vi "New SPL Calc.vi"(10 "Filtered Signal":dynamicdata(waveform), 11 "Reset":bool) -> (3 "SPL Out":dbl)   [LabVIEW 2020, in "CollectionSupport.lvlib"]
uses:
  CollectionSupport.lvlib
  <vilib>/measure/madcrms.llb/Basic Averaged DC-RMS for 1 Chan.vi
  <vilib>/measure/NI_MAPro.lvlib
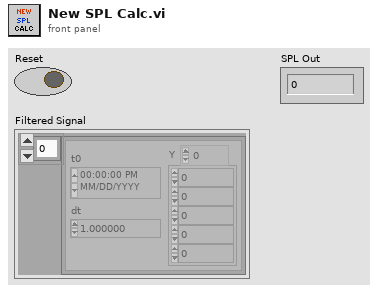
[diagram p1: front panel]
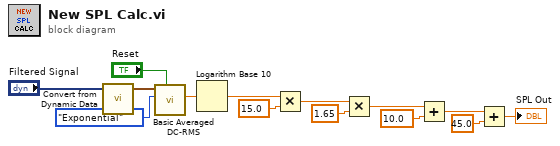
[diagram p0: block diagram]
diagram:
  n1 = call "Convert from Dynamic Data"("Dynamic Data Type"="Filtered Signal") -> ("Waveform"=w11:waveform(dbl))  [unwired: 3 in]
  n2 = call-poly <vilib>:"Basic Averaged DC-RMS.vi"("reset"="Reset", "averaging type"=enum16{"Linear", "Exponential"}."Exponential", "signal in"=w11) -> ("RMS value"=w1:dbl)  [unwired: 5 in, 3 out]
  n3 = Logarithm Base 10(1:w1) -> (0:w7:dbl)
  n4 = Multiply(x=w7, y=15.0) -> (x*y=w6:dbl)
  n5 = Multiply(x=w6, y=1.65) -> (x*y=w4:dbl)
  n6 = Add(x=w4, y=10.0) -> (x+y=w9:dbl)
  n7 = Add(x=w9, y=45.0) -> (x+y=→"SPL Out":dbl)
